vi "Initialize.vi"(5 "Password":string, 7 "Username":string, 8 "error in (no error)":errorcluster, 10 "Address":string, 11 "SCP File Transfer in":refnum<class "SCP File Transfer.lvclass">) -> (0 "error out":errorcluster, 3 "SCP File Transfer out":refnum<class "SCP File Transfer.lvclass">)   [LabVIEW 2013, in "PL Framework Configuration Tool.lvlib" / "SCP File Transfer.lvclass"]
doc: "Initializes a specific file transfer protocol session for the given target based upon the specific implementation class passed in."
uses:
  SCP File Transfer.lvclass
  SCP File Transfer.lvclass/SCP File Transfer.ctl
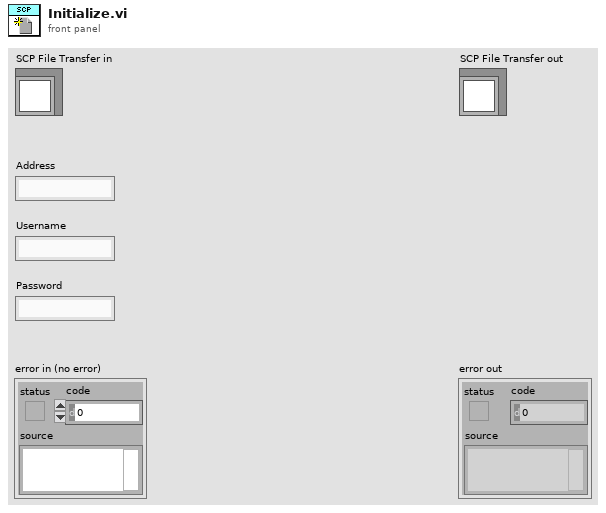
[diagram p1: front panel]
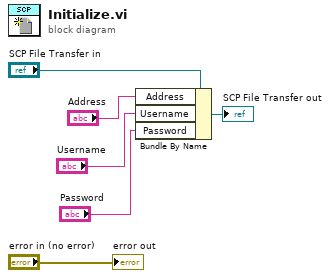
[diagram p0: block diagram]
diagram:
  n1 = Bundle By Name(cluster="SCP File Transfer in", "Address"="Address", "Username"="Username", "Password"="Password") -> (→"SCP File Transfer out":refnum<class "SCP File Transfer.lvclass">)
  "error out" <- "error in (no error)"
